vi "Compute Centroid.vi"(8 "Input Valid":bool, 9 "Image Height":u16, 10 "Image Width":u16, 11 "Pixel":bool) -> (0 "Output valid":bool, 2 "Y":fxp<+,32,16>, 3 "X":fxp<+,32,16>)   [LabVIEW 2012]
doc: "This VI computes the centroid of a binary image. It is intended to be run on an FPGA."
uses:
  <vilib>/rvi/FXPMathLib/FxpDiv/subVIs/nifxpmath_Div_SimConfig.ctl
  <vilib>/rvi/FXPMathLib/FxpDiv/simVIs/DllFxpDivTemp_sub.vi
  <vilib>/rvi/FXPMathLib/FxpDiv/XNode/nifxpmath_Div.xnode
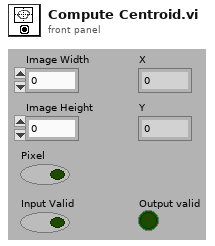
[diagram p1: front panel]
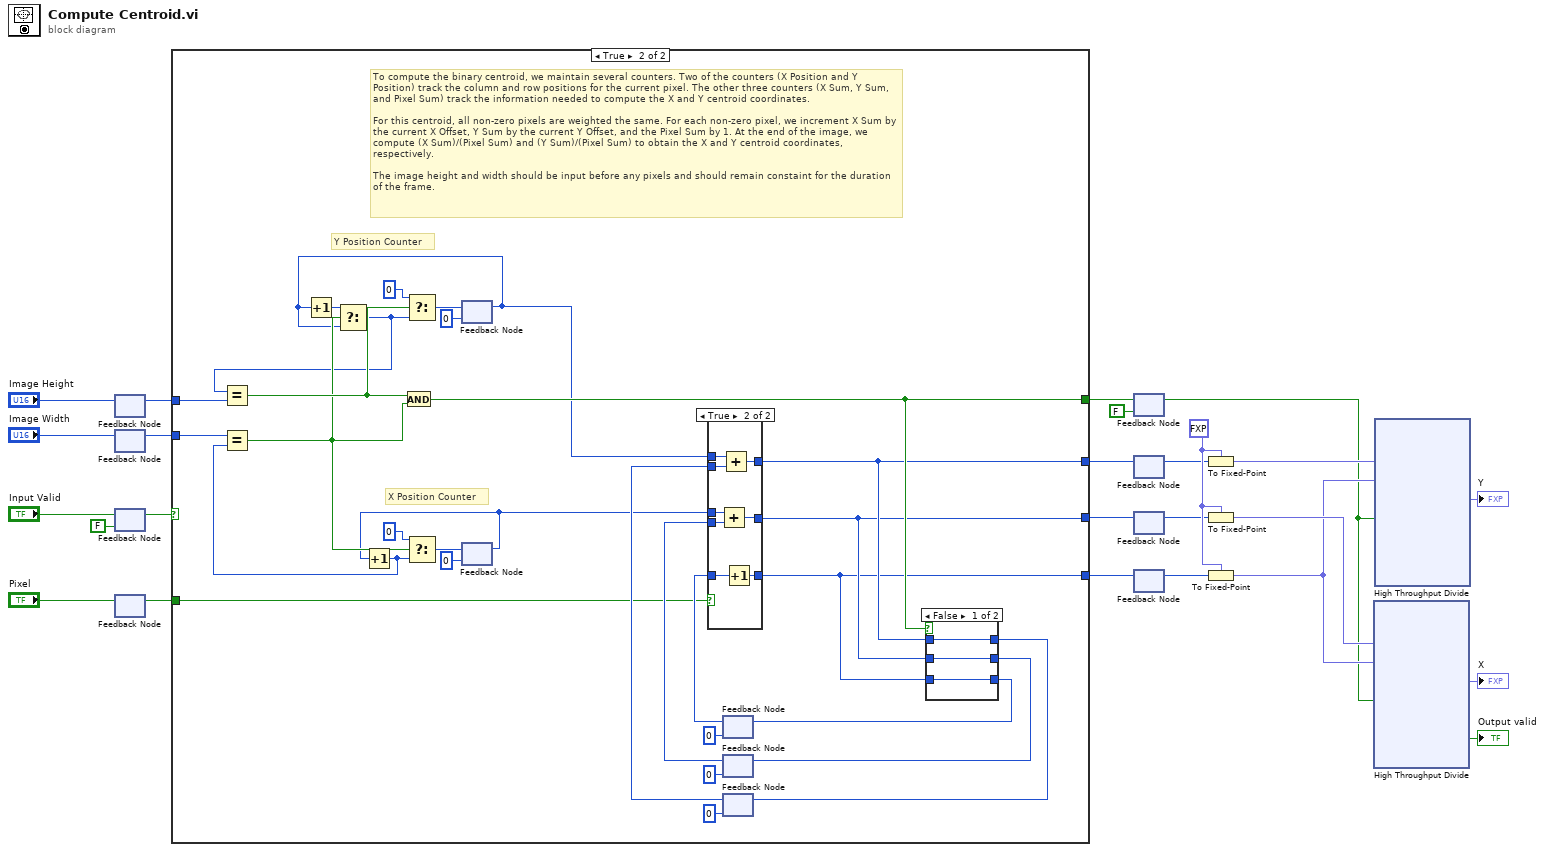
[diagram p0: block diagram]
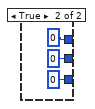
[diagram p3: hidden frame]
diagram:
  w14 = fxp<+,32,32> 0.0 ("fixed-point type")
  n1 = feedback #1() -> (w20:u16)  [unwired: 1 in]
  n2 = feedback-in #1("Image Height") -> ()
  n3 = feedback #2() -> (w19:u16)  [unwired: 1 in]
  n4 = feedback-in #2("Image Width") -> ()
  n5 = feedback #3(FALSE ("Input Valid")) -> (w21:bool)
  n6 = feedback-in #3("Input Valid") -> ()
  n7 = feedback #4() -> (w18:bool)  [unwired: 1 in]
  n8 = feedback-in #4("Pixel") -> ()
  n9 = case shown="True" w21 {
    tunnel: [_ w43] -> w9
    tunnel: w20 -> [_ w37]
    tunnel: w19 -> [_ w32]
    tunnel: w18 -> [_ w38]
    tunnel: [_ w30] -> w6
    tunnel: [_ w29] -> w7
    tunnel: [_ w28] -> w8
    frame False {
      # "If the input is not valid, then do not update the accumulators."
    }
    frame True {
      # "To compute the binary centroid, we maintain several counters. Two of the counters (X Position and Y Position) track the column and row positions for the current pixel. The other three counters (X Sum, Y Sum, and Pixel Sum) track the information needed to compute the X and Y centroid coordinates.\n\nFor this centroid, all non-zero pixels are weighted the same. For each non-zero pixel, we increment X Sum by the current X Offset, Y Sum by the current Y Offset, and the Pixel Sum by 1. At the end of the image, we compute (X Sum)/(Pixel Sum) and (Y Sum)/(Pixel Sum) to obtain the X and Y centroid coordinates, respectively.\n\nThe image height and width should be input before any pixels and should remain constaint for the duration of the frame."
      # "X Position Counter"
      # "Y Position Counter"
      n10 = feedback #5(u16 0 ("t")) -> (w26:u16)
      n11 = Increment(x=w26) -> (x+1=w35:u16)
      n12 = feedback #6(u16 0 ("t")) -> (w27:u16)
      n13 = Increment(x=w27) -> (x+1=w31:u16)
      n14 = Equal?(x=w32, y=w31) -> (x = y?=w47:bool)
      n15 = Select(t=w35, s=w47, f=w26) -> (s? t:f=w34:u16)
      n16 = Equal?(x=w34, y=w37) -> (x = y?=w50:bool)
      n17 = And(x=w50, y=w47) -> (x .and. y?=w43:bool)
      n18 = Select(t=u16 0, s=w50, f=w34) -> (s? t:f=w40:u16)
      n19 = Select(t=u16 0, s=w47, f=w31) -> (s? t:f=w42:u16)
      n20 = feedback-in #5(w40) -> ()
      n21 = feedback-in #6(w42) -> ()
      n22 = feedback #7(u32 0 ("Pixel 0")) -> (w45:u32)
      n23 = feedback #8(u32 0 ("Pixel 0")) -> (w54:u32)
      n24 = feedback #9(u32 0 ("Pixel 0")) -> (w53:u32)
      n25 = case shown="True" w38 {
        tunnel: [w63 w71] -> w29
        tunnel: w54 -> [w63 w70]
        tunnel: w53 -> [w62 w69]
        tunnel: [w62 w68] -> w30
        tunnel: w27 -> [_ w67]
        tunnel: w26 -> [_ w66]
        tunnel: [w61 w65] -> w28
        tunnel: w45 -> [w61 w64]
        frame False {
        }
        frame True {
          n26 = Add(x=w67, y=w70) -> (x+y=w71:u32)
          n27 = Add(x=w66, y=w69) -> (x+y=w68:u32)
          n28 = Increment(x=w64) -> (x+1=w65:u32)
        }
      }
      n29 = case shown="False" w43 {
        tunnel: w29 -> [w56 _]
        tunnel: [w56 u32 0 ("Pixel 0")] -> w49
        tunnel: w30 -> [w57 _]
        tunnel: [w57 u32 0 ("Pixel 0")] -> w48
        tunnel: w28 -> [w55 _]
        tunnel: [w55 u32 0 ("Pixel 0")] -> w46
        frame False {
        }
        frame True {
        }
      }
      n30 = feedback-in #7(w46) -> ()
      n31 = feedback-in #8(w49) -> ()
      n32 = feedback-in #9(w48) -> ()
    }
  }
  n33 = feedback-in #10(w9) -> ()
  n34 = feedback #10(FALSE) -> (w2:bool)
  n35 = feedback #11() -> (w5:u32)  [unwired: 1 in]
  n36 = feedback-in #11(w6) -> ()
  n37 = feedback #12() -> (w4:u32)  [unwired: 1 in]
  n38 = feedback-in #12(w7) -> ()
  n39 = feedback #13() -> (w3:u32)  [unwired: 1 in]
  n40 = feedback-in #13(w8) -> ()
  n41 = To Fixed-Point(fixed-point type=w14, number=w5) -> (fixed-point=w13:fxp<+,32,32>)
  n42 = To Fixed-Point(fixed-point type=w14, number=w4) -> (fixed-point=w12:fxp<+,32,32>)
  n43 = To Fixed-Point(fixed-point type=w14, number=w3) -> (fixed-point=w11:fxp<+,32,32>)
  n44 = xnode "High Throughput Divide"("x"=w12, "y"=w11, "input valid"=w2) -> ("x/y"=→"X":fxp<+,32,16>, "output valid"=→"Output valid":bool)  [unwired: 1 in, 1 out]
  n45 = xnode "High Throughput Divide"("x"=w13, "y"=w11, "input valid"=w2) -> ("x/y"=→"Y":fxp<+,32,16>)  [unwired: 1 in, 2 out]
